vi "Trig_Function.vi"() -> ()   [LabVIEW 2022 SP3]
panel:
  out "Tangent":dbl
  out "Cosine":dbl
  out "Sine":dbl format="%.2f"
  in  "Angle in Radians":dbl
  # "Trig_Function\nEnter any rational number into the field below. The sine, cosine, and tangent of that angle will be calculated."
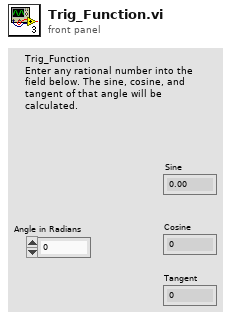
[diagram p1: front panel]
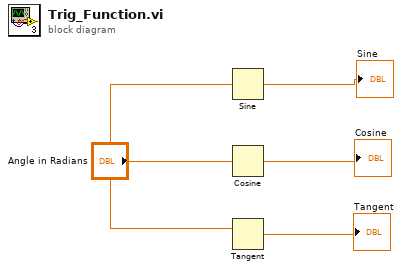
[diagram p0: block diagram]
diagram:
  n1 = Sine(x="Angle in Radians") -> (sin(x)=→"Sine":dbl)
  n2 = Cosine(x="Angle in Radians") -> (cos(x)=→"Cosine":dbl)
  n3 = Tangent(1:"Angle in Radians") -> (0:→"Tangent":dbl)
